vi "Move.vi"() -> ()   [LabVIEW 2013]
uses:
  <vilib>/Instr/_visa.llb/VISA Configure Serial Port (Instr).vi
panel:
  in  "Time":u16=2000 max=30000 step=1
  in  "Angel":dbl min=0.0 max=240.0 step=0.24
  out "error out":errorcluster
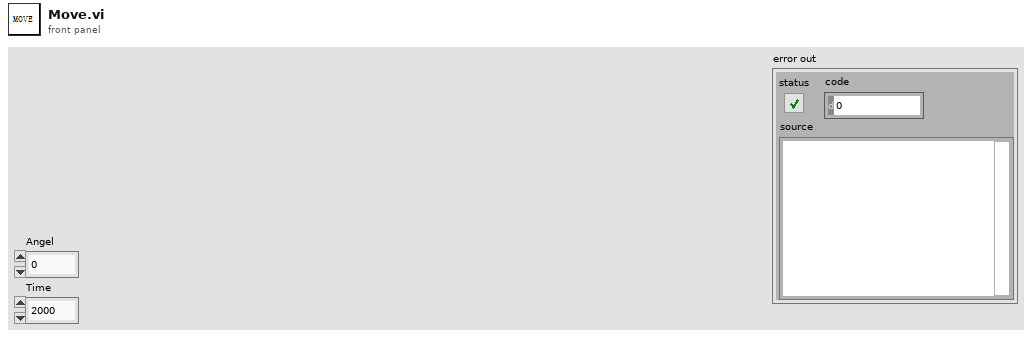
[diagram p1: front panel]
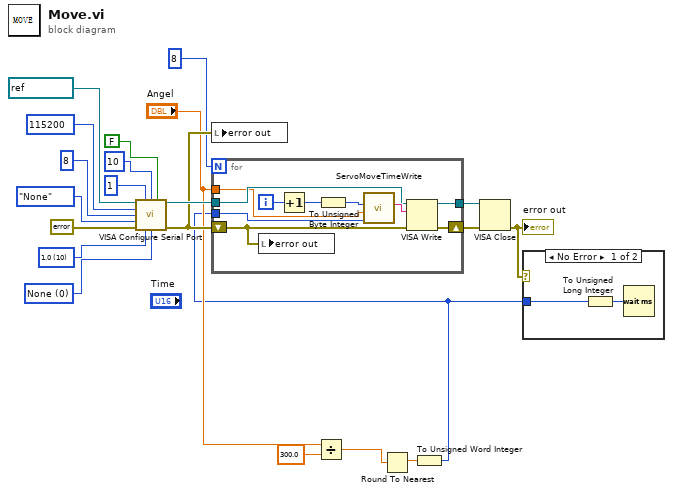
[diagram p0: block diagram]
diagram:
  w16 = u16 0 items=["None", "XON/XOFF", "RTS/CTS", "XON/XOFF & RTS/CTS", "DTR/DSR", "XON/XOFF & DTR/DSR"] ("flow control (0:none)")
  w17 = u16 10 items=["1.0"=10, "1.5"=15, "2.0"=20] ("stop bits (10: 1 bit)")
  n1 = call-poly "VISA Configure Serial Port"("VISA resource name"=refnum<visa-resource-name> "COM7", "timeout (10sec)"=u32 1, "termination char\n(0xA = '\\n' = LF)"=u8 10 ("termination char\n(0xA = '\\n' = LF)"), "Enable Termination\nChar (T)"=FALSE ("Enable Termination\nChar (T)"), "baud rate (9600)"=u32 115200, "data bits (8)"=u16 8, "parity (0:none)"=enum16{"None", "Odd", "Even", "Mark", "Space"}."None", "error in (no error)"=errorcluster {"status"=FALSE, "code"=0, "source"=""}, "stop bits (10: 1 bit)"=w17, "flow control (0:none)"=w16) -> ("VISA resource name out"=w11:refnum<visa-resource-name>, "error out"=w10:errorcluster)  [unwired: 4 in]
  n2 = local write "error out"(w10) -> ()
  n3 = Divide(x="Angel", y=300.0) -> (x/y=w3:dbl)
  n4 = Round To Nearest(number=w3) -> (nearest integer value=w2:dbl)
  n5 = To Unsigned Word Integer(number=w2) -> (unsigned 16bit integer=w1:u16)
  n6 = for {
    N: 8 -> [_]
    shift-right: [w26] -> w9
    shift-left: w10 -> [w24]
    tunnel: w11 -> [w27]
    tunnel: [w25] -> w8
    tunnel: "Angel" -> [w23]
    tunnel: w1 -> [w22]
    i -> [w31]
    n7 = local write "error out"(w24) -> ()
    n8 = Increment(x=w31) -> (x+1=w29:i32)
    n9 = To Unsigned Byte Integer(number=w29) -> (unsigned 8bit integer=w30:u8)
    n10 = call "ServoMoveTimeWrite.vi"("Time"=w22, "Angel"=w23, "ID"=w30) -> ("Command"=w28:string)  [unwired: 8 in]
    n11 = VISA Write(VISA resource name=w27, write buffer=w28, error in (no error)=w24) -> (VISA resource name out=w25:refnum<visa-resource-name>, error out=w26:errorcluster)  [unwired: 1 out]
  }
  n12 = VISA Close(VISA resource name=w8, error in (no error)=w9) -> (error out=w6:errorcluster)
  "error out" <- w6
  n13 = case shown="No Error" w6 {
    tunnel: w1 -> [w33 _]
    frame No Error {
      n14 = To Unsigned Long Integer(number=w33) -> (unsigned 32bit integer=w32:u32)
      n15 = Wait (ms)(milliseconds to wait=w32) -> ()  [unwired: 1 out]
    }
    frame Error {
    }
  }
